vi "StartGUI.vi"(8 "Error In":errorcluster, 11 "reference in":refnum<class "MasterGUI.lvclass">) -> (0 "Error Out":errorcluster, 3 "reference in":refnum<class "MasterGUI.lvclass">)   [LabVIEW 2021, in "MasterGUI.lvclass"]
uses:
  MasterGUI.lvclass
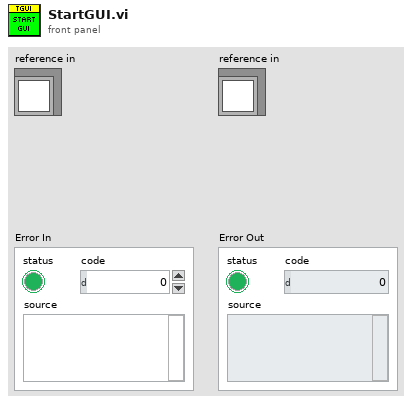
[diagram p1: front panel]
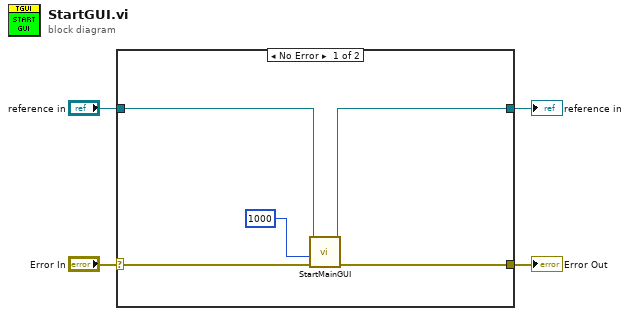
[diagram p0: block diagram]
diagram:
  n1 = case shown="No Error" "Error In" {
    selector: "Error In" -> [w9 w11]
    tunnel: [w8 w11] -> w3
    tunnel: [w7 w10] -> w1
    tunnel: "reference in" -> [w6 w10]
    frame No Error {
      n2 = call "StartMainGUI.vi"("Error In"=w9, "ms timeout (-1)"=1000, "reference in"=w6) -> ("Error Out"=w8:errorcluster, "reference out"=w7:refnum<class "MasterGUI.lvclass">)  [unwired: 5 in, 2 out]
    }
    frame Error {
    }
  }
  "Error Out" <- w3
  "reference in" <- w1
